vi "2D Array Decimate.vi"(8 "averaging":bool=TRUE, 9 "y decimating factor":dbl=1.0, 10 "x decimating factor":dbl=1.0, 11 "Input 2D Array":dbl[][](array[numeric])) -> (1 "y dim":u32, 2 "x dim":u32, 3 "output array":dbl[][](array[numeric]))   [LabVIEW 2018]
uses:
  <vilib>/Analysis/2dsp.llb/Decimate (single shot, DBL).vi
  <vilib>/Analysis/NI_AALPro.lvlib
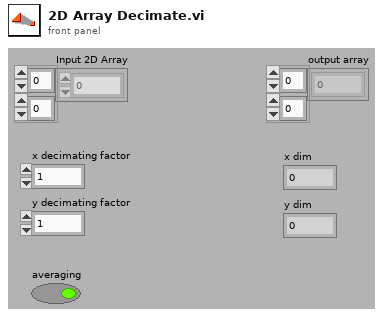
[diagram p1: front panel]
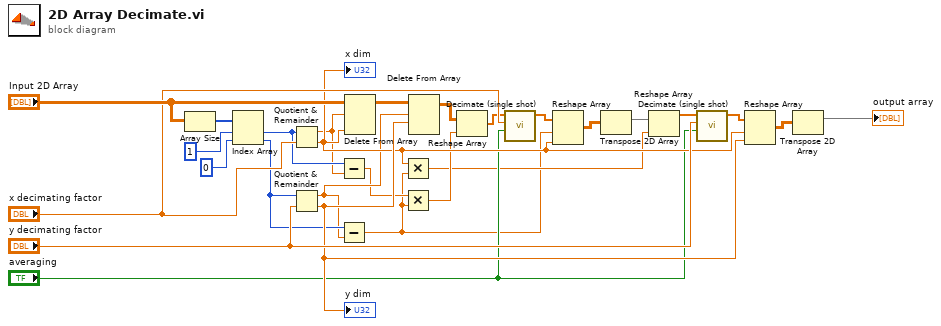
[diagram p0: block diagram]
diagram:
  n1 = Array Size(array="Input 2D Array") -> (size(s)=w10:i32[])
  n2 = Index Array(array=w10, index #1=1 ("index"), index #2=0 ("index")) -> (element #1=w7:i32, element #2=w5:i32)
  n3 = Quotient & Remainder(x=w7, y="x decimating factor") -> (x-y*floor(x/y)=w6:dbl, floor(x/y)=w23:dbl)
  "x dim" <- w23
  n4 = Quotient & Remainder(x=w5, y="y decimating factor") -> (x-y*floor(x/y)=w4:dbl, floor(x/y)=w24:dbl)
  "y dim" <- w24
  n5 = Subtract(x=w7, y=w6) -> (x-y=w3:dbl)
  n6 = Subtract(x=w5, y=w4) -> (x-y=w2:dbl)
  n7 = Delete From Array(array="Input 2D Array", length=w6, index (col)=w23) -> (array with subset deleted=w8:dbl[][])  [unwired: 1 in, 1 out]
  n8 = Multiply(x=w23, y=w2) -> (x*y=w12:dbl)
  n9 = Multiply(x=w3, y=w2) -> (x*y=w15:dbl)
  n10 = Delete From Array(array=w8, length=w4, index (row)=w24) -> (array with subset deleted=w9:dbl[][])  [unwired: 1 in, 1 out]
  n11 = Reshape Array(w9, w15) -> (w16:dbl[])
  n12 = call-poly <vilib>:"Decimate (single shot).vi"("averaging"="averaging", "decimating factor"="x decimating factor", "X"=w16) -> ("Decimated Array"=w1:dbl[])  [unwired: 8 out]
  n13 = Reshape Array(w1, w2, w23) -> (w19:dbl[][])
  n14 = Transpose 2D Array(2D array=w19) -> (transposed array=w14:dbl[][])
  n15 = Reshape Array(w14, w12) -> (w18:dbl[])
  n16 = call-poly <vilib>:"Decimate (single shot).vi"("averaging"="averaging", "decimating factor"="y decimating factor", "X"=w18) -> ("Decimated Array"=w17:dbl[])  [unwired: 8 out]
  n17 = Reshape Array(w17, w23, w24) -> (w13:dbl[][])
  n18 = Transpose 2D Array(2D array=w13) -> (transposed array=→"output array":dbl[][])
